vi "LogErrorCheckPoint.vi"(0 "GenericCanAdapterClass in":refnum<class "GenericCanAdapterClass.lvclass">, 1 "LogSuspend":bool, 11 "error in":errorcluster) -> (4 "GenericCanAdapterClass out":refnum<class "GenericCanAdapterClass.lvclass">, 15 "error out":errorcluster)   [LabVIEW 2011, in "GenericCanAdapterClass.lvclass"]
uses:
  GenericCanAdapterClass.lvclass
  GenericCanAdapterClass.lvclass/GenericCanAdapterClass.ctl
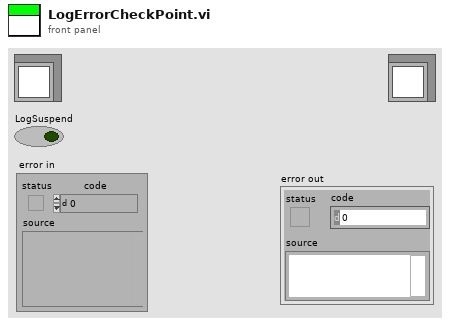
[diagram p1: front panel]
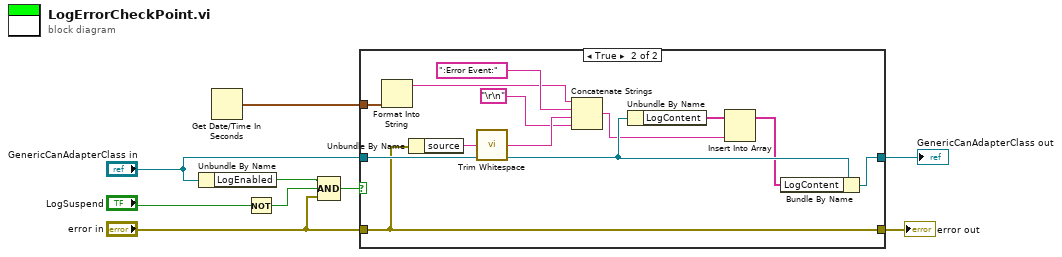
[diagram p0: block diagram]
diagram:
  n1 = Unbundle By Name("GenericCanAdapterClass in") -> ("LogEnabled"=w6:bool)
  n2 = Get Date/Time In Seconds() -> (seconds since 1Jan1904=w7:timestamp)
  n3 = Not(x="LogSuspend") -> (.not. x?=w4:bool)
  n4 = Compound Arithmetic op=AND(w6, w4, "error in") -> (w5:bool)
  n5 = case shown="True" w5 {
    tunnel: "error in" -> [w11 w15]
    tunnel: [w11 w15] -> w9
    tunnel: [w10 w23] -> w1
    tunnel: "GenericCanAdapterClass in" -> [w10 w22]
    tunnel: w7 -> [_ w21]
    frame False {
    }
    frame True {
      n6 = Format Into String(w21) -> (resulting string=w16:string)  [unwired: 3 in, 1 out]
      n7 = Unbundle By Name(w15) -> ("source"=w19:string)
      n8 = call <vilib>:"Trim Whitespace.vi"("string"=w19) -> ("trimmed string"=w20:string)  [unwired: 1 in]
      n9 = Concatenate Strings(w16, ":Error Event:" ("string"), w20, "\r\n") -> (w13:string)
      n10 = Unbundle By Name(w22) -> ("LogContent"=w14:string[])
      n11 = Insert Into Array(array=w14, new element=w13) -> (w12:string[])  [unwired: 1 in]
      n12 = Bundle By Name(cluster=w22, "LogContent"=w12) -> (w23:refnum<class "GenericCanAdapterClass.lvclass">)
    }
  }
  "error out" <- w9
  "GenericCanAdapterClass out" <- w1
